vi "TimedLoop-Tune.vi"(0 "Late":bool, 5 "dt In":i64, 7 "T (ms)":dbl, 11 "State In":T1) -> (6 "dt Out":i64, 15 "State Out":T1)   [LabVIEW 2020]
uses:
  TimedLoop-Tuning State.ctl
panel:
  in  "Max late":i32=5
  in  "Max dt":i64=20
  in  "Max late rate (/10s)":dbl
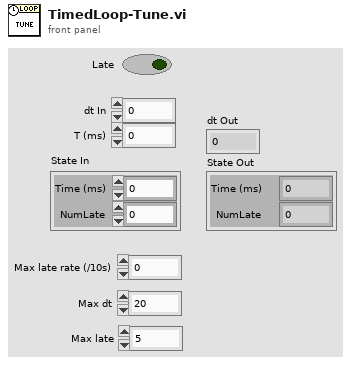
[diagram p1: front panel]
types:
  T1 = typedef "TimedLoop-Tuning State.ctl" = cluster{"Time (ms)":dbl, "NumLate":i32}
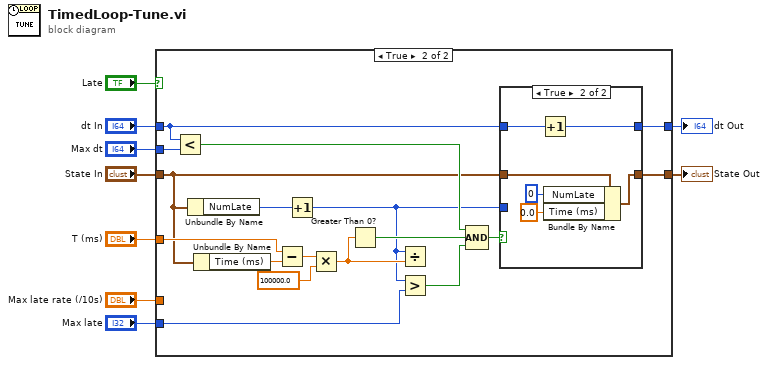
[diagram p0: block diagram]
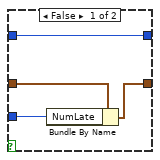
[diagram p3: hidden frame]
diagram:
  n1 = case shown="True" "Late" {
    tunnel: "State In" -> [w10 w19]
    tunnel: "T (ms)" -> [_ w27]
    tunnel: "Max late rate (/10s)" -> [_ _]
    tunnel: "dt In" -> [w11 w22]
    tunnel: "Max dt" -> [_ w24]
    tunnel: [w11 w21] -> w3
    tunnel: [w10 w20] -> w2
    tunnel: "Max late" -> [_ w13]
    frame False {
    }
    frame True {
      n2 = Less?(x=w22, y=w24) -> (x < y?=w23:bool)
      n3 = Unbundle By Name(w19) -> ("NumLate"=w28:i32)
      n4 = Unbundle By Name(w19) -> ("Time (ms)"=w18:dbl)
      n5 = Subtract(x=w27, y=w18) -> (x-y=w26:dbl)
      n6 = Increment(x=w28) -> (x+1=w15:i32)
      n7 = Multiply(x=w26, y=100000.0) -> (x*y=w16:dbl)
      n8 = Greater Than 0?(x=w16) -> (x > 0?=w17:bool)
      n9 = Divide(x=w15, y=w16) -> ()  [unwired: 1 out]
      n10 = Greater?(x=w15, y=w13) -> (0:w14:bool)
      n11 = Compound Arithmetic op=AND(w23, w17, w14) -> (w12:bool)
      n12 = case shown="True" w12 {
        tunnel: w22 -> [w32 w38]
        tunnel: w19 -> [w31 w36]
        tunnel: [w32 w37] -> w21
        tunnel: [w30 w33] -> w20
        tunnel: w15 -> [w29 _]
        frame False {
          n13 = Bundle By Name(cluster=w31, "NumLate"=w29) -> (w30:T1)
        }
        frame True {
          n14 = Increment(x=w38) -> (x+1=w37:i64)
          n15 = Bundle By Name(cluster=w36, "NumLate"=0, "Time (ms)"=0.0) -> (w33:T1)
        }
      }
    }
  }
  "dt Out" <- w3
  "State Out" <- w2
